vi "start.vi"(8 "error in (no error)":errorcluster, 11 "CameraNetworkController in":refnum<class "CameraNetworkController.lvclass">) -> (0 "error out":errorcluster, 3 "CameraNetworkController out":refnum<class "CameraNetworkController.lvclass">)   [LabVIEW 2009, in "Hardware.lvlib" / "HWControllers.lvlib" / "CameraNetworkController.lvclass"]
uses:
  CameraNetworkController.lvclass
  NetworkClient/NetworkServer.lvclass
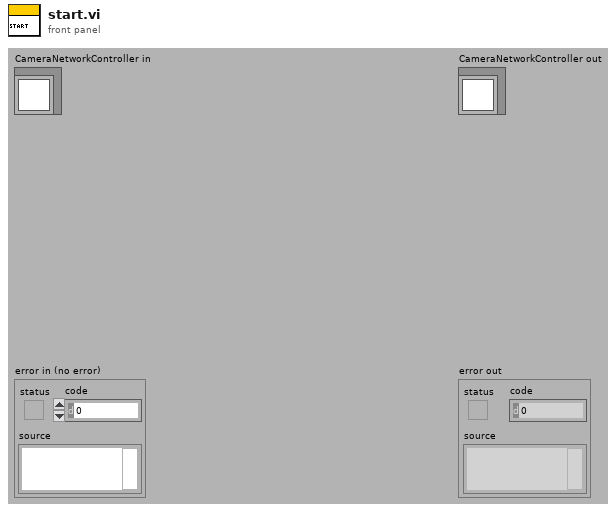
[diagram p1: front panel]
types:
  T1 = cluster{"Message":enum16{"Idle", "initialise", "configureAcquisition", "setTemperature", "getTemperature", "start", "stop", "sendImage", "close", "error", "ExitApp"}, "Data":variant}
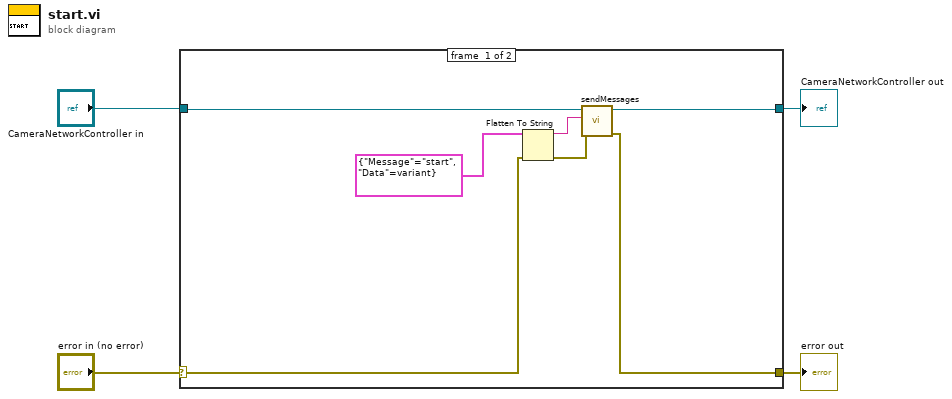
[diagram p0: block diagram]
diagram:
  n1 = case shown="No Error" "error in (no error)" {
    selector: "error in (no error)" -> [w6 w13]
    tunnel: [w5 w13] -> w3
    tunnel: [w9 w12] -> w1
    tunnel: "CameraNetworkController in" -> [w8 w12]
    frame #0 {
      n2 = Flatten To String(anything=T1 {"Message"=enum."start", "Data"=variant}, error in (no error)=w6) -> (data string=w10:string, error out=w11:errorcluster)  [unwired: 3 out]
      n3 = call "sendMessages.vi"("error in (no error)"=w11, "messageString"=w10, "NetworkClient in"=w8) -> ("error out"=w5:errorcluster, "NetworkClient out"=w9:refnum<class "CameraNetworkController.lvclass">)  [unwired: 7 in]
    }
    frame #1 {
    }
  }
  "error out" <- w3
  "CameraNetworkController out" <- w1
